vi "Open.vi"(8 "error in (no error)":errorcluster, 11 "Serial Port":string) -> (0 "error out":errorcluster, 3 "FW102C out":i32, 5 "Connected?":bool)   [LabVIEW 2018, in "Thorlabs_FW102C.lvlib"]
uses:
  Thorlabs_FW102C.lvlib
  E:/Program Files (x86)/National Instruments/LabVIEW 2011/instr.lib/Thorlabs_FW102C/Library/FilterWheel102_win32.dll
  Library/FilterWheel102_win64.dll
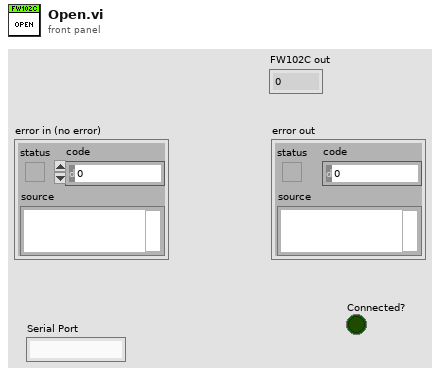
[diagram p1: front panel]
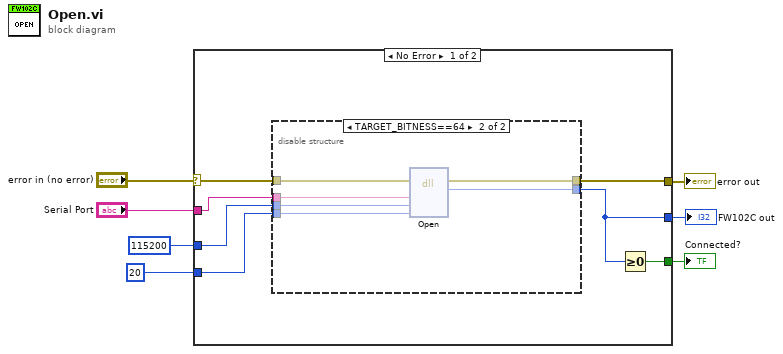
[diagram p0: block diagram]
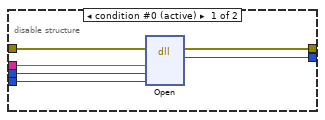
[diagram p2: hidden frame]
diagram:
  n1 = case shown="No Error" "error in (no error)" {
    selector: "error in (no error)" -> [w14 w27]
    tunnel: [w13 w27] -> w6
    tunnel: 20 ("timeout") -> [w11 _]
    tunnel: "Serial Port" -> [w12 _]
    tunnel: [w9 _] -> w3
    tunnel: [w8 _] -> w2
    tunnel: 115200 ("nbaud") -> [w10 _]
    frame No Error {
      n2 = disable-structure shown="TARGET_BITNESS==64" {
        disable-tunnel: w14 -> [w20 w26]
        disable-tunnel: [w19 w25] -> w13
        disable-tunnel: w12 -> [w18 w24]
        disable-tunnel: w11 -> [w17 w23]
        disable-tunnel: w10 -> [w16 w22]
        disable-tunnel: [w15 w21] -> w8
        frame condition #0 (active) {
          n3 = dll-call lib="E:/Program Files (x86)/National Instruments/LabVIEW 2011/instr.lib/Thorlabs_FW102C/Library/FilterWheel102_win32.dll" fn="Open"(error in=w20, "Serial No"=w18, "nBaud"=w16, "timeout"=w17) -> (error out=w19:errorcluster, "hdl"=w15:i32)  [unwired: 5 in, 1 out]
        }
        frame condition #1 {
          n4 = dll-call lib="C:/Users/aspitarl/Git/MHDLab/Filter Wheel/Thorlabs_FW102C/Library/FilterWheel102_win64.dll" fn="Open"(error in=w26, "Serial No"=w24, "nBaud"=w22, "timeout"=w23) -> (error out=w25:errorcluster, "hdl"=w21:i32)  [unwired: 5 in, 1 out]
        }
      }
      n5 = Greater Or Equal To 0?(x=w8) -> (x >= 0?=w9:bool)
    }
    frame Error {
    }
  }
  "error out" <- w6
  "Connected?" <- w3
  "FW102C out" <- w2
